vi "Revision Query.vi"(8 "error in (no error)":errorcluster, 11 "MC switch refnum in":refnum<k24>) -> (0 "error out":errorcluster, 1 "Instrument Firmware Revision":string, 2 "Instrument Driver Revision":string, 3 "MC switch refnum out":refnum<k24>)   [LabVIEW 2019, in "Minicircuit RF Switch Box.lvlib"]
doc: "Queries the current instrument firmware revision and instrument driver revision."
uses:
  <instrlib>/LV_Minicircuit_RF_Switch/Minicircuit RF Switch Box.lvlib
  C:/Program Files (x86)/National Instruments/LabVIEW 2019/instr.lib/LV_Minicircuit_RF_Switch/mcl_RF_Switch_Controller_NET45.dll
  mcl_RF_Switch_Controller_NET45.dll
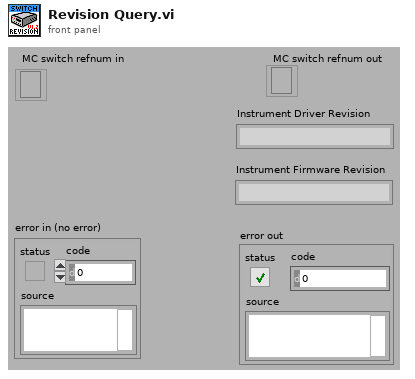
[diagram p1: front panel]
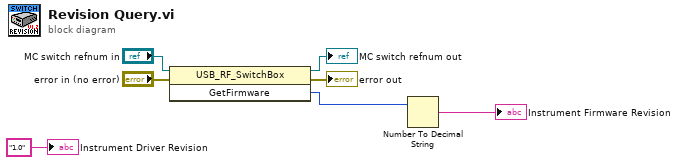
[diagram p0: block diagram]
diagram:
  n1 = invoke class="USB_RF_SwitchBox" method="GetFirmware"(reference="MC switch refnum in", error in="error in (no error)") -> (reference out=→"MC switch refnum out":refnum<k24>, error out=→"error out":errorcluster, "GetFirmware"=w3:i32)  [unwired: 1 in]
  n2 = Number To Decimal String(number=w3) -> (decimal integer string=→"Instrument Firmware Revision":string)  [unwired: 1 in]
  "Instrument Driver Revision" <- "1.0" ("Instrument Driver Revision")
